vi "Bristol Wavemeter.vi"() -> ()   [LabVIEW 2012]
uses:
  Libraries and VIs/CLDevIFace.dll
panel:
  out "Lambda Off Read (nm)":dbl=828.2984734786044 format="%.5f"
  in  "Bristol In":i32=5
  out "Bristol Out":i32=4
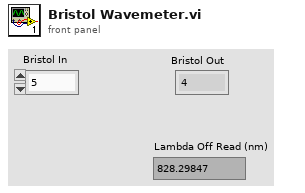
[diagram p1: front panel]
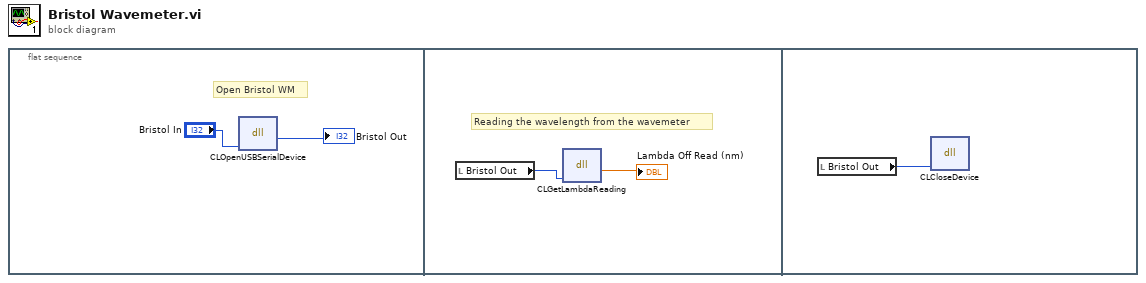
[diagram p0: block diagram]
diagram:
  n1 = flat-sequence {
    frame #0 {
      # "Open Bristol WM"
      n2 = dll-call lib="C:/Users/H2ODial/Desktop/Shared Telescope WV DIAL Code/Libraries and VIs/CLDevIface.dll" fn="CLOpenUSBSerialDevice"("commPort"="Bristol In") -> ("return type"=→"Bristol Out":i32)  [unwired: 4 in, 2 out]
    }
    frame #1 {
      # "Reading the wavelength from the wavemeter"
      n3 = local read "Bristol Out"() -> (w3:i32)
      n4 = dll-call lib="C:/Users/H2ODial/Desktop/Shared Telescope WV DIAL Code/Libraries and VIs/CLDevIface.dll" fn="CLGetLambdaReading"("devHandle"=w3) -> ("return type"=→"Lambda Off Read (nm)":dbl)  [unwired: 4 in, 2 out]
    }
    frame #2 {
      n5 = local read "Bristol Out"() -> (w5:i32)
      n6 = dll-call lib="C:/Users/H2ODial/Desktop/Shared Telescope WV DIAL Code/Libraries and VIs/CLDevIface.dll" fn="CLCloseDevice"("devHandle"=w5) -> ()  [unwired: 5 in, 2 out]
    }
  }
